vi "SaveTestLog.vi"(10 "output array 3":string[][](array[string])) -> (2 "String 2":string)   [LabVIEW 2013]
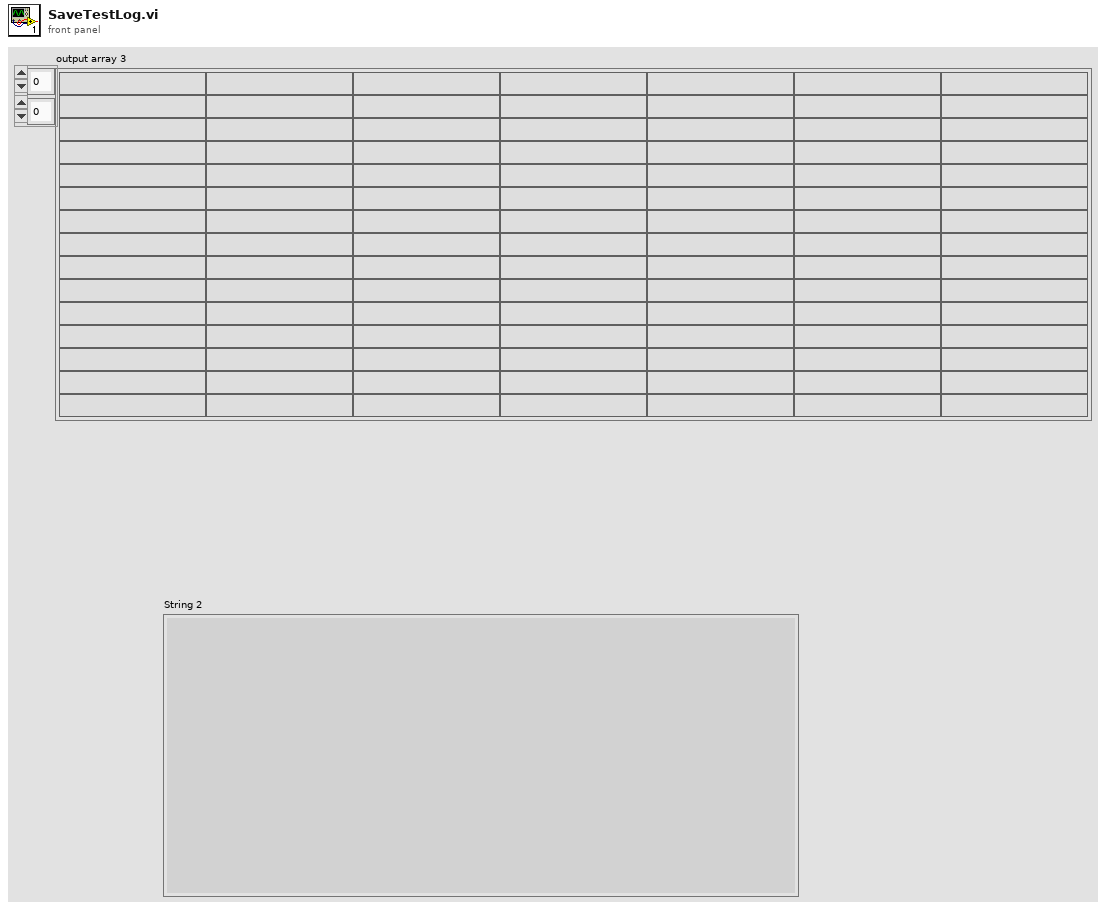
[diagram p1: front panel]
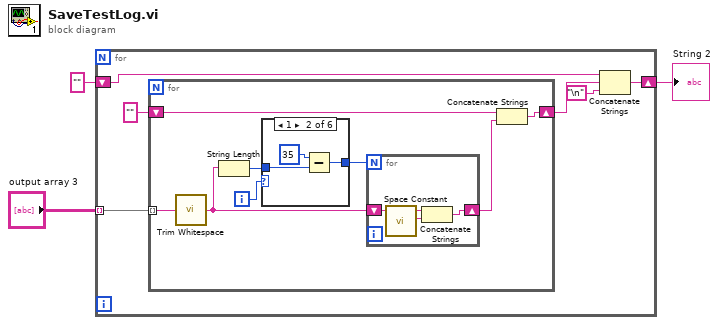
[diagram p0: block diagram]
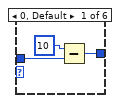
[diagram p2: hidden frame]
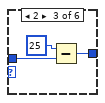
[diagram p3: hidden frame]
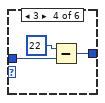
[diagram p4: hidden frame]
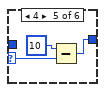
[diagram p5: hidden frame]
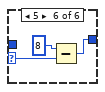
[diagram p6: hidden frame]
diagram:
  n1 = for {
    tunnel: "output array 3" -> [w9] mode=indexing
    shift-right: [w6] -> w1
    shift-left: "" -> [w7]
    n2 = for {
      tunnel: w9 -> [w17] mode=indexing
      shift-right: [w15] -> w5
      shift-left: "" -> [w16]
      i -> [w14]
      n3 = call <vilib>:"Trim Whitespace.vi"("string"=w17) -> ("trimmed string"=w12:string)  [unwired: 1 in]
      n4 = String Length(string=w12) -> (length=w13:i32)
      n5 = case shown="1" w14 {
        selector: w14 -> [_ _ _ _ w35 w38]
        tunnel: w13 -> [w22 w26 w29 w32 _ _]
        tunnel: [w21 w25 w27 w30 w33 w36] -> w11
        frame 0, Default {
          n6 = Subtract(x=10, y=w22) -> (x-y=w21:i32)
        }
        frame 1 {
          n7 = Subtract(x=35, y=w26) -> (x-y=w25:i32)
        }
        frame 2 {
          n8 = Subtract(x=25, y=w29) -> (x-y=w27:i32)
        }
        frame 3 {
          n9 = Subtract(x=22, y=w32) -> (x-y=w30:i32)
        }
        frame 4 {
          n10 = Subtract(x=10, y=w35) -> (x-y=w33:i32)
        }
        frame 5 {
          n11 = Subtract(x=8, y=w38) -> (x-y=w36:i32)
        }
      }
      n12 = for {
        N: w11 -> [_]
        shift-right: [w19] -> w10
        shift-left: w12 -> [w20]
        n13 = call <vilib>:"Space Constant.vi"() -> ("String"=w18:string)
        n14 = Concatenate Strings(w20, w18) -> (w19:string)
      }
      n15 = Concatenate Strings(w16, w10) -> (w15:string)
    }
    n16 = Concatenate Strings(w7, w5, "\n") -> (w6:string)
  }
  "String 2" <- w1
